vi "MEMR-Compute Noise Floor.vi"(0 "State In":T2, 5 "Analysis":T1, 7 "Avg":dbl[][](array[numeric]), 9 "Npts":i32) -> (4 "Noise spectra":cluster{"Freq (Hz)":dbl[], "Mag (dB)":dbl[]}[](array[cluster]))   [LabVIEW 2015]
uses:
  Typedefs/MEMR-Analysis State.ctl
  MEMR-Offline Analysis Parameters.ctl
  Typedefs/MEMR-Analysis.ctl
  PXI DAQ VIs/Utility VIs/Array Dimensions (2D).vi
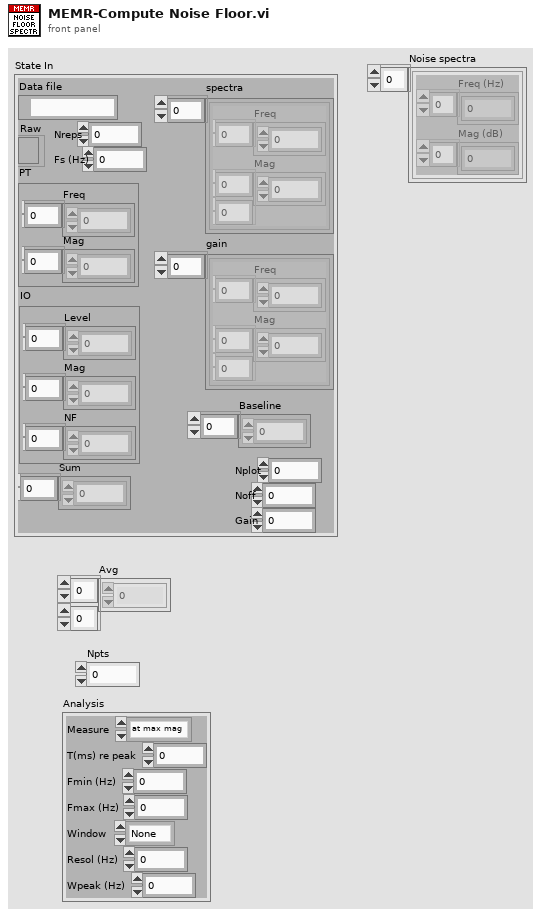
[diagram p1: front panel]
types:
  T1 = typedef "MEMR-Offline Analysis Parameters.ctl" = cluster{"Measure":enum16{"at max mag", "at max gain", "over window", "optimize"}, "T(ms) re peak":dbl, "Fmin (Hz)":dbl, "Fmax (Hz)":dbl, "Window":enum16{"None", "Hanning", "Hamming"}, "Resol (Hz)":dbl, "Wpeak (Hz)":dbl}
  T2 = typedef "MEMR-Analysis State.ctl" = cluster{"Data file":path, "Raw":refnum<file>, "PT":cluster{"Freq":dbl[], "Mag":dbl[]}, "IO":cluster{"Level":dbl[], "Mag":dbl[], "NF":dbl[]}, "Nreps":i32, "Fs (Hz)":dbl, "Sum":dbl[], "Nplot":i32, "Noff":i32, "Gain":dbl, "spectra":cluster{"Freq":dbl[], "Mag":dbl[][]}[], "gain":cluster{"Freq":dbl[], "Mag":dbl[][]}[], "Baseline":dbl[]}
  T3 = typedef "MEMR-Analysis.ctl" = cluster{"T(ms) re peak":dbl, "Fmin (Hz)":dbl, "Fmax (Hz)":dbl, "Window":enum16{"None", "Hanning", "Hamming"}, "Gain (dB)":dbl, "Resol (Hz)":dbl}
  T4 = cluster{"Freq (Hz)":dbl[], "+Freq. Mag of FFT (dB rms)":dbl[]}
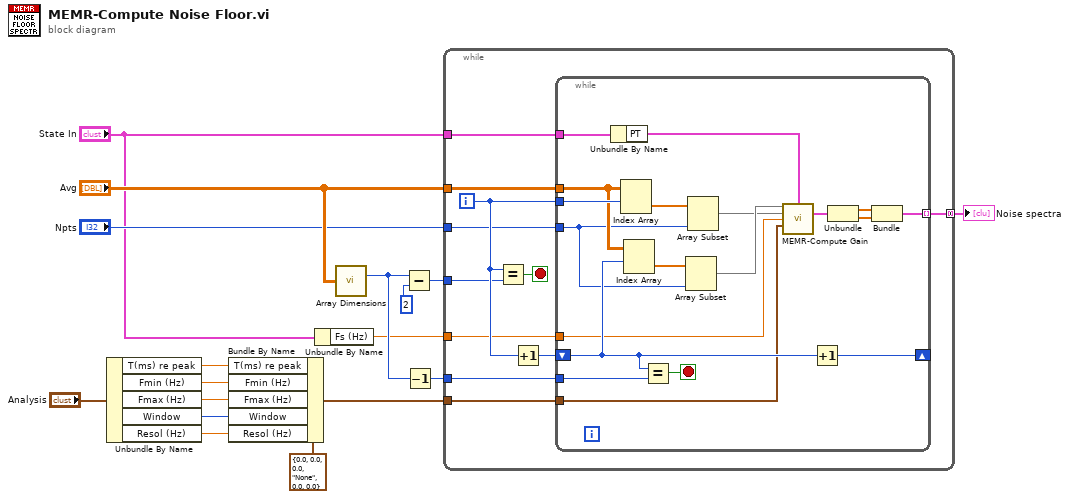
[diagram p0: block diagram]
diagram:
  n1 = Unbundle By Name("Analysis") -> ("T(ms) re peak"=w6:dbl, "Fmin (Hz)"=w5:dbl, "Fmax (Hz)"=w4:dbl, "Window"=w3:enum16{"None", "Hanning", "Hamming"}, "Resol (Hz)"=w2:dbl)
  n2 = Bundle By Name(cluster=T3 {"T(ms) re peak"=0.0, "Fmin (Hz)"=0.0, "Fmax (Hz)"=0.0, "Window"=enum."None", "Gain (dB)"=0.0, "Resol (Hz)"=0.0} ("Analysis"), "T(ms) re peak"=w6, "Fmin (Hz)"=w5, "Fmax (Hz)"=w4, "Window"=w3, "Resol (Hz)"=w2) -> (w1:T3)
  n3 = Unbundle By Name("State In") -> ("Fs (Hz)"=w10:dbl)
  n4 = call-poly "Array Dimensions.vi"("2D Array"="Avg") -> ("# rows"=w13:i32)  [unwired: 13 in, 1 out]
  n5 = Subtract(x=w13, y=2) -> (x-y=w17:i32)
  n6 = Decrement(x=w13) -> (x-1=w12:i32)
  n7 = while {
    tunnel: "State In" -> [w28]
    tunnel: "Avg" -> [w27]
    tunnel: w1 -> [w26]
    tunnel: w17 -> [w18]
    tunnel: "Npts" -> [w22]
    tunnel: w12 -> [w21]
    tunnel: w10 -> [w20]
    tunnel: [w19] -> w9 mode=concatenating
    i -> [w24]
    stop <- w25 stop-if-true
    n8 = Equal?(x=w24, y=w18) -> (x = y?=w25:bool)
    n9 = Increment(x=w24) -> (x+1=w23:i32)
    n10 = while {
      tunnel: w28 -> [w38]
      tunnel: w27 -> [w44]
      tunnel: w26 -> [w36]
      tunnel: w24 -> [w47]
      shift-right: [w45] -> _
      shift-left: w23 -> [w43]
      tunnel: w22 -> [w40]
      tunnel: w21 -> [w39]
      tunnel: w20 -> [w35]
      tunnel: [w33] -> w19 mode=indexing
      stop <- w46 stop-if-true
      n11 = Unbundle By Name(w38) -> ("PT"=w37:cluster{"Freq":dbl[], "Mag":dbl[]})
      n12 = Index Array(array=w44, index (row)=w47) -> (element=w41:dbl[])  [unwired: 1 in]
      n13 = Index Array(array=w44, index (row)=w43) -> (element=w42:dbl[])  [unwired: 1 in]
      n14 = Equal?(x=w43, y=w39) -> (x = y?=w46:bool)
      n15 = Array Subset(array=w42, length=w40) -> (w31:dbl[])  [unwired: 1 in]
      n16 = Array Subset(array=w41, length=w40) -> (w30:dbl[])  [unwired: 1 in]
      n17 = call "MEMR-Compute Gain.vi"("Test"=w31, "PT"=w37, "Baseline"=w30, "Fs (Hz)"=w35, "Analysis"=w36) -> ("gain spectrum"=w34:T4)  [unwired: 8 in, 2 out]
      n18 = Increment(x=w43) -> (x+1=w45:i32)
      n19 = Unbundle(w34) -> ("Freq (Hz)"=w32:dbl[], "+Freq. Mag of FFT (dB rms)"=w29:dbl[])
      n20 = Bundle("Freq (Hz)"=w32, "+Freq. Mag of FFT (dB rms)"=w29) -> (w33:T4)  [unwired: 1 in]
    }
  }
  "Noise spectra" <- w9
